vi "Corr Digitizer Reload.vi"(8 "error in (no error)":errorcluster, 11 "digitizer corrections in":T1) -> (0 "error out":errorcluster, 3 "digitizer corrections out":T1)   [LabVIEW 2020]
doc: "Takes correction path from the correction session and tries to load the digitizer corrections file. If the path is empty it will clear all the correction data in the correction session (blank correction)."
uses:
  Corr Digitizers.ctl
  octave/infolib/GetString.vi
  octave/infolib/Get 1D String.vi
  <vilib>/Utility/error.llb/Error Cluster From Error Code.vi
  <vilib>/ErrorRing/Error Ring.xnode
  octave/infolib/infolib.lvlib
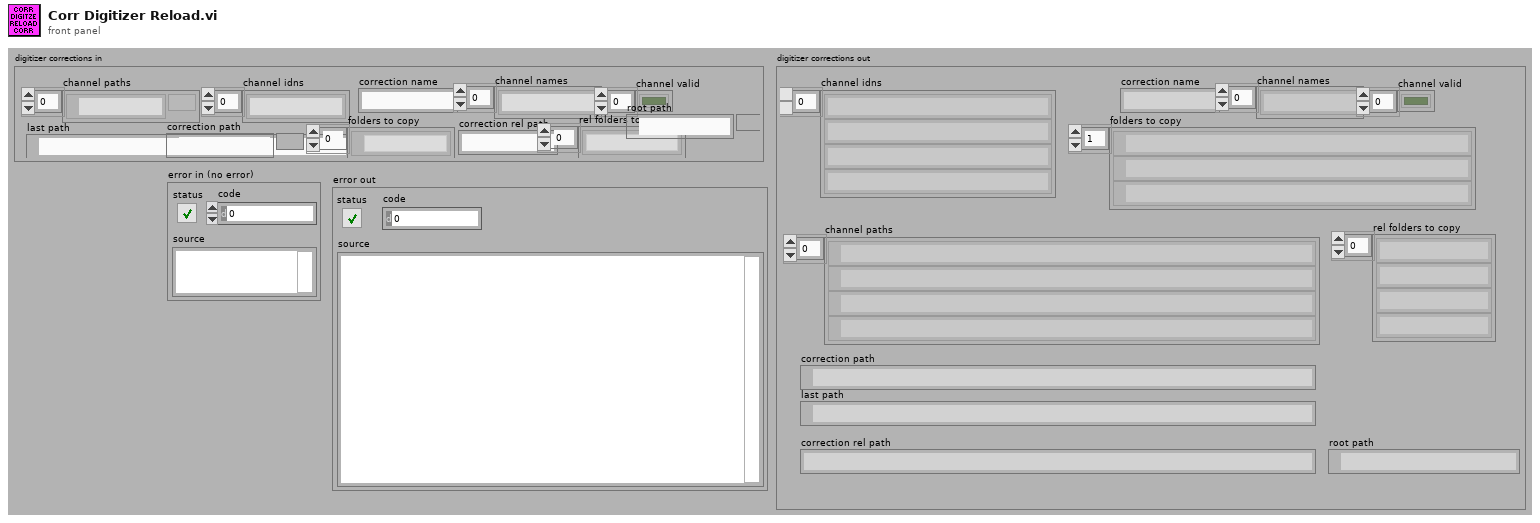
[diagram p1: front panel]
types:
  T1 = typedef "Corr Digitizers.ctl" = cluster{"last path":path, "channel paths":path[], "channel idns":string[], "correction name":string, "channel names":string[], "folders to copy":path[], "channel valid":bool[], "correction path":path, "correction rel path":string, "rel folders to copy":string[], "root path":path}
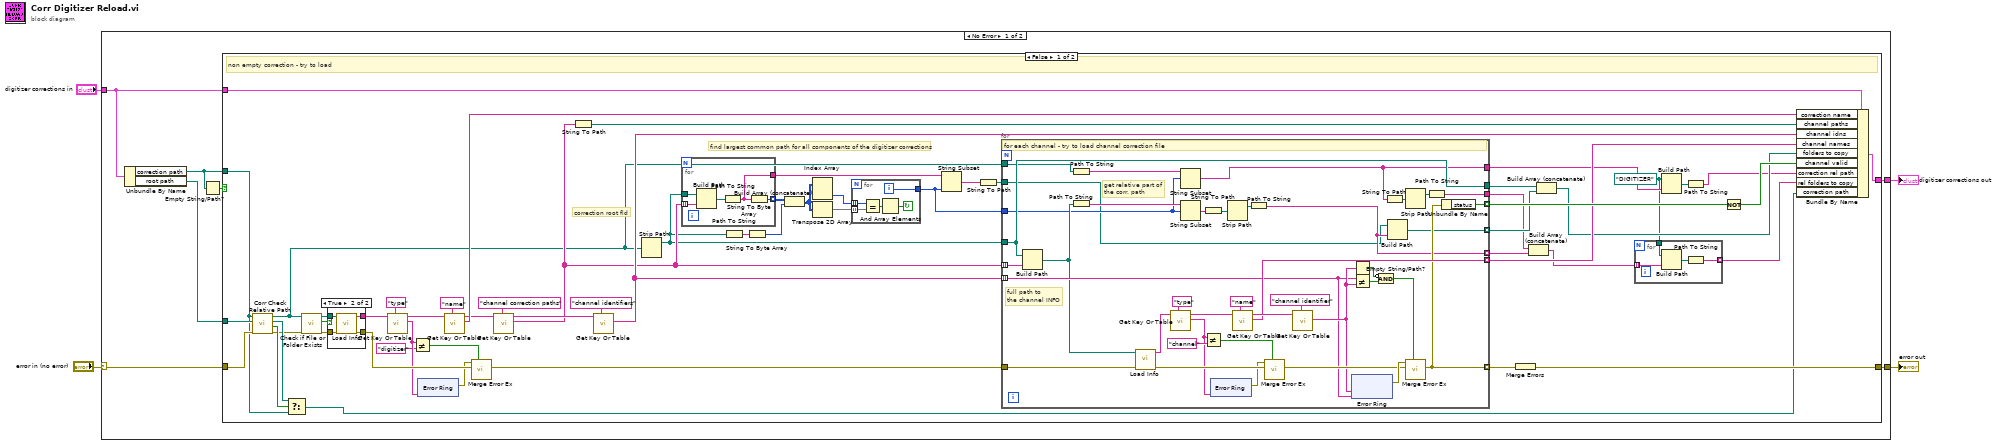
[diagram p0: block diagram]
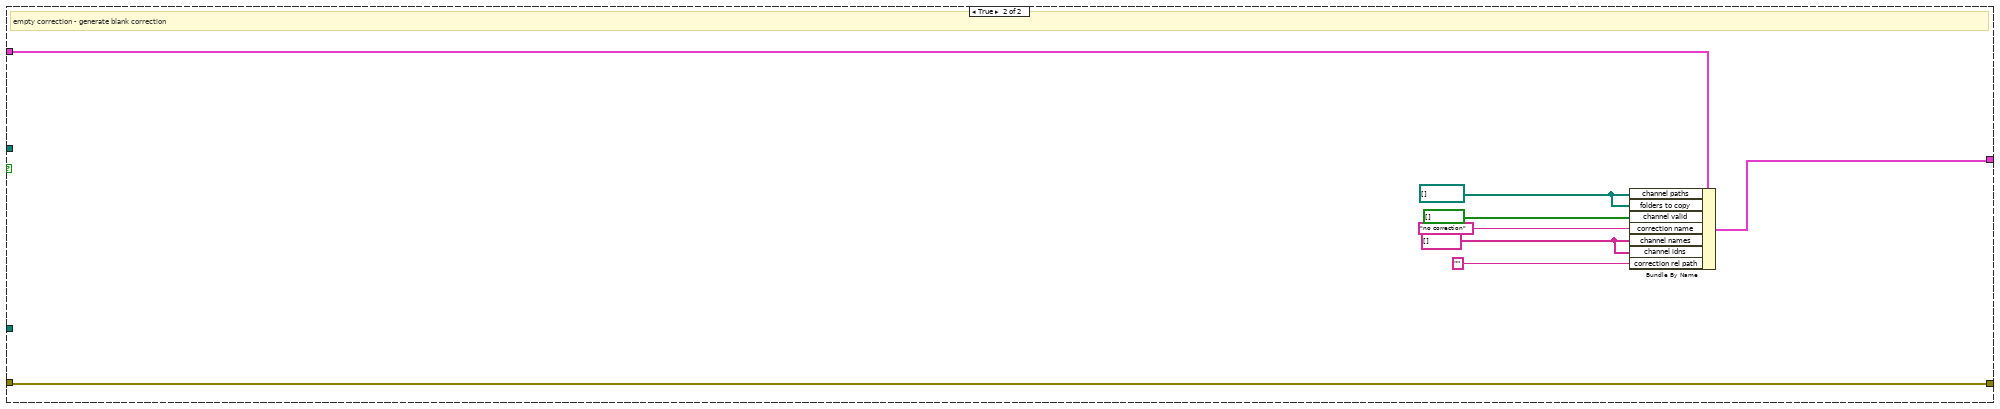
[diagram p3: hidden frame]
diagram:
  n1 = case shown="No Error" "error in (no error)" {
    selector: "error in (no error)" -> [w8 w158]
    tunnel: [w11 w158] -> w4
    tunnel: [w10 w159] -> w3
    tunnel: "digitizer corrections in" -> [w9 w159]
    frame No Error {
      n2 = Unbundle By Name(w9) -> ("correction path"=w6:path, "root path"=w5:path)
      n3 = Empty String/Path?(string/path=w6) -> (empty?=w7:bool)
      n4 = case shown="False" w7 {
        tunnel: [w69 w157] -> w11
        tunnel: [w68 w152] -> w10
        tunnel: w9 -> [w46 w156]
        tunnel: w6 -> [w22 _]
        tunnel: w8 -> [w26 w157]
        tunnel: w5 -> [w25 _]
        frame False {
          w28 = path "DIGITIZER" ("base path")
          # "find largest common path for all components of the digitizer corrections"
          # "correction root fld"
          # "non empty correction - try to load"
          n5 = call "Corr Check Relative Path.vi"("error in"=w26, "root path"=w25, "input path"=w22) -> ("error out"=w20:errorcluster, "relative path valid?"=w24:bool, "relative path"=w23:path, "absolute path"=w13:path)  [unwired: 4 in, 1 out]
          n6 = Select(t=w23, s=w24, f=w22) -> (s? t:f=w21:path)
          n7 = call <vilib>:"Check if File or Folder Exists.vi"("error in (no error)"=w20, "path"=w13) -> ("error out"=w19:errorcluster, "file or folder exists?"=w17:bool, "dup path"=w18:path)  [unwired: 7 in]
          n8 = case shown="True" w17 {
            tunnel: [w70 w74] -> w60
            tunnel: [_ w73] -> w47
            tunnel: w19 -> [w70 w72]
            tunnel: w18 -> [_ w71]
            frame False {
            }
            frame True {
              n9 = call "Load Info.vi"("error in"=w72, "filename"=w71) -> ("error out"=w74:errorcluster, "info data"=w73:string)  [unwired: 8 in]
            }
          }
          n10 = call-poly "Get Key Or Table.vi"("key description"="type", "info data"=w47) -> ("value"=w51:string, "info data out"=w53:string)  [unwired: 6 in, 2 out]
          n11 = Not Equal?(x=w51, y="digitizer") -> (x != y?=w52:bool)
          n12 = xnode "Error Ring"("parameter 0"=w51) -> ("error out"=w50:errorcluster)
          n13 = call-poly "Get Key Or Table.vi"("key description"="name", "info data"=w53) -> ("value"=w58:string, "info data out"=w55:string)  [unwired: 6 in, 2 out]
          n14 = call "Merge Error Ex.vi"("Is error? (False)"=w52, "main error in (no error)"=w60, "second error in"=w50) -> ("error out"=w61:errorcluster)  [unwired: 8 in]
          n15 = call-poly "Get Key Or Table.vi"("key description"="channel correction paths", "info data"=w55) -> ("value"=w41:string[], "info data out"=w59:string)  [unwired: 6 in, 2 out]
          n16 = String To Path(string=w41) -> (path=w62:path[])
          n17 = call-poly "Get Key Or Table.vi"("key description"="channel identifiers", "info data"=w59) -> ("value"=w63:string[])  [unwired: 6 in, 3 out]
          n18 = Strip Path(path=w13) -> (stripped path=w12:path)  [unwired: 1 out]
          n19 = for {
            tunnel: w12 -> [w79]
            tunnel: w41 -> [w78] mode=indexing
            tunnel: [w76] -> w40
            tunnel: [w77] -> w39 mode=indexing
            n20 = Build Path(base path=w79, name or relative path=w78) -> (appended path=w75:path)
            n21 = Path To String(path=w75) -> (string=w76:string)
            n22 = String To Byte Array(string=w76) -> (unsigned byte array=w77:u8[])
          }
          n23 = Path To String(path=w12) -> (string=w38:string)
          n24 = String To Byte Array(string=w38) -> (unsigned byte array=w37:u8[])
          n25 = Build Array (concatenate)(w39, w37) -> (w14:u8[][])
          n26 = Index Array(array=w14) -> (element=w15:u8[])  [unwired: 2 in]
          n27 = Transpose 2D Array(2D array=w14) -> (transposed array=w16:u8[][])
          n28 = for {
            tunnel: w16 -> [w91] mode=indexing
            tunnel: [w88] -> w34
            tunnel: w15 -> [w87] mode=indexing
            i -> [w88]
            stop <- w89 continue-if-true
            n29 = Equal?(x=w87, y=w91) -> (x = y?=w90:bool[])
            n30 = And Array Elements(Boolean array=w90) -> (logical AND=w89:bool)
          }
          n31 = String Subset(string=w40, length (rest)=w34) -> (substring=w36:string)  [unwired: 1 in]
          n32 = String To Path(string=w36) -> (path=w35:path)
          n33 = for {
            tunnel: w61 -> [w134]
            tunnel: w12 -> [w110]
            tunnel: w41 -> [w133] mode=indexing
            tunnel: w63 -> [w114] mode=indexing
            tunnel: [w119] -> w65 mode=indexing
            tunnel: [w113] -> w64 mode=indexing
            tunnel: [w112] -> w66 mode=indexing
            tunnel: [w111] -> w44 mode=indexing
            tunnel: [w110] -> w45
            tunnel: [w109] -> w31
            tunnel: w13 -> [w97]
            tunnel: [w106] -> w43
            tunnel: [w102] -> w42 mode=indexing
            tunnel: w35 -> [w96]
            tunnel: w34 -> [w99]
            # "get relative part of\nthe corr. path"
            # "full path to\nthe channel INFO"
            # "for each channel - try to load channel correction file"
            n34 = Build Path(base path=w110, name or relative path=w133) -> (appended path=w101:path)
            n35 = Path To String(path=w97) -> (string=w98:string)
            n36 = Path To String(path=w101) -> (string=w100:string)
            n37 = call "Load Info.vi"("error in"=w134, "filename"=w101) -> ("error out"=w129:errorcluster, "info data"=w132:string)  [unwired: 8 in]
            n38 = call-poly "Get Key Or Table.vi"("key description"="type", "info data"=w132) -> ("value"=w126:string, "info data out"=w125:string)  [unwired: 6 in, 2 out]
            n39 = String Subset(string=w98, offset (0)=w99) -> (substring=w109:string)  [unwired: 1 in]
            n40 = String Subset(string=w100, offset (0)=w99) -> (substring=w105:string)  [unwired: 1 in]
            n41 = String To Path(string=w105) -> (path=w104:path)
            n42 = Not Equal?(x=w126, y="channel") -> (x != y?=w127:bool)
            n43 = xnode "Error Ring"("parameter 0"=w126) -> ("error out"=w128:errorcluster)
            n44 = Strip Path(path=w104) -> (stripped path=w103:path)  [unwired: 1 out]
            n45 = call-poly "Get Key Or Table.vi"("key description"="name", "info data"=w125) -> ("value"=w119:string, "info data out"=w122:string)  [unwired: 6 in, 2 out]
            n46 = Path To String(path=w103) -> (string=w102:string)
            n47 = call "Merge Error Ex.vi"("Is error? (False)"=w127, "main error in (no error)"=w129, "second error in"=w128) -> ("error out"=w117:errorcluster)  [unwired: 8 in]
            n48 = call-poly "Get Key Or Table.vi"("key description"="channel identifier", "info data"=w122) -> ("value"=w115:string)  [unwired: 6 in, 3 out]
            n49 = xnode "Error Ring"("parameter 0"=w115, "parameter 1"=w114) -> ("error out"=w118:errorcluster)
            n50 = Empty String/Path?(string/path=w115) -> (empty?=w120:bool)
            n51 = Not Equal?(x=w114, y=w115) -> (x != y?=w121:bool)
            n52 = Compound Arithmetic op=AND(invert w120, w121) -> (w116:bool)
            n53 = String To Path(string=w109) -> (path=w108:path)
            n54 = Build Path(base path=w96, name or relative path=w102) -> (appended path=w111:path)
            n55 = call "Merge Error Ex.vi"("Is error? (False)"=w116, "main error in (no error)"=w117, "second error in"=w118) -> ("error out"=w113:errorcluster)  [unwired: 8 in]
            n56 = Strip Path(path=w108) -> (stripped path=w107:path)  [unwired: 1 out]
            n57 = Path To String(path=w107) -> (string=w106:string)
            n58 = Unbundle By Name(w113) -> ("status"=w112:bool)
          }
          n59 = Merge Errors(w64) -> (w69:errorcluster)
          n60 = Build Array (concatenate)(w43, w42) -> (w29:string[])
          n61 = Build Array (concatenate)(w45, w44) -> (w33:path[])
          n62 = for {
            tunnel: w29 -> [w93] mode=indexing
            tunnel: w28 -> [w94]
            tunnel: [w92] -> w27 mode=indexing
            n63 = Build Path(base path=w94, name or relative path=w93) -> (appended path=w95:path)
            n64 = Path To String(path=w95) -> (string=w92:string)
          }
          n65 = Build Path(base path=w28, name or relative path=w31) -> (appended path=w32:path)
          n66 = Path To String(path=w32) -> (string=w30:string)
          n67 = Not(x=w66) -> (.not. x?=w67:bool[])
          n68 = Bundle By Name(cluster=w46, "correction name"=w58, "channel paths"=w62, "channel idns"=w63, "channel names"=w65, "folders to copy"=w33, "channel valid"=w67, "correction rel path"=w30, "rel folders to copy"=w27, "correction path"=w21) -> (w68:T1)
        }
        frame True {
          w151 = string[] [] ("channel names")
          w155 = path[] [] ("channel paths")
          # "empty correction - generate blank correction"
          n69 = Bundle By Name(cluster=w156, "channel paths"=w155, "folders to copy"=w155, "channel valid"=bool[] [], "correction name"="no correction", "channel names"=w151, "channel idns"=w151, "correction rel path"="") -> (w152:T1)
        }
      }
    }
    frame Error {
    }
  }
  "error out" <- w4
  "digitizer corrections out" <- w3
